vi "LOGGER.vi"() -> ()   [LabVIEW 2015]
panel:
  in  "file path (use dialog) 2":path
  in  "Boolean":bool
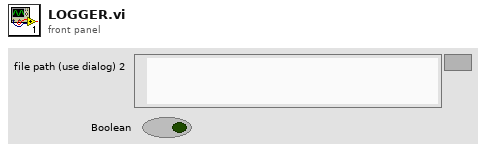
[diagram p1: front panel]
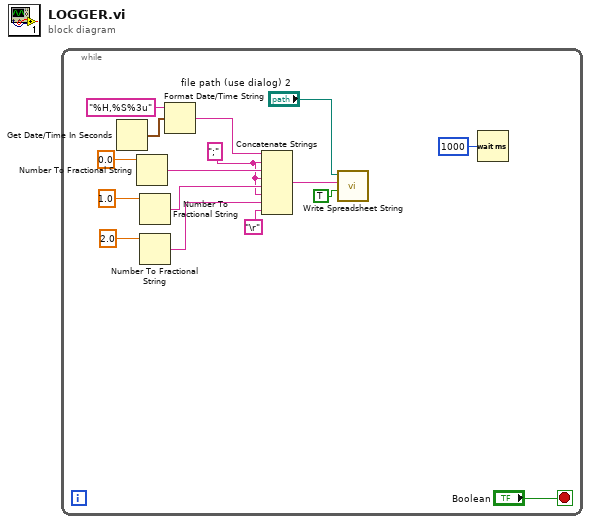
[diagram p0: block diagram]
diagram:
  n1 = while {
    stop <- "Boolean" stop-if-true
    w3 = ";" ("delimiter (\\t)")
    n2 = Get Date/Time In Seconds() -> (seconds since 1Jan1904=w10:timestamp)
    n3 = Number To Fractional String(number=0.0) -> (F-format string=w5:string)  [unwired: 3 in]
    n4 = Number To Fractional String(number=1.0) -> (F-format string=w4:string)  [unwired: 3 in]
    n5 = Number To Fractional String(number=2.0) -> (F-format string=w2:string)  [unwired: 3 in]
    n6 = Format Date/Time String(time format string (%c)="%H,%S%3u", seconds (now)=w10) -> (date/time string=w9:string)  [unwired: 1 in]
    n7 = Concatenate Strings(w9, w3, w5, w3, w4, w3, w2, "\r") -> (w15:string)
    n8 = call <vilib>:"Write Spreadsheet String.vi"("append to file? (new file:F)"=TRUE, "spreadsheet string"=w15, "file path (dialog if empty)"="file path (use dialog) 2") -> ()  [unwired: 7 in, 2 out]
    n9 = Wait (ms)(milliseconds to wait=u32 1000) -> ()  [unwired: 1 out]
  }
